vi "Filter by Favorites.vi"(8 "error in (no error)":errorcluster, 10 "Favorites? (T)":bool=TRUE, 11 "Contacts":T1[](array[typedef])) -> (0 "error out":errorcluster, 3 "Filtered Contacts":T1[](array[typedef]))   [LabVIEW 2014, in "Contact Data.lvlib"]
doc: "Filters an array of contacts to only include favorites or to not include favorites."
uses:
  Contact Data.lvlib
  Control Sort Mode.ctl
  Position.ctl
  Contact.ctl
  Controls.ctl
  DesinationControls.ctl
  DestinationCluster.ctl
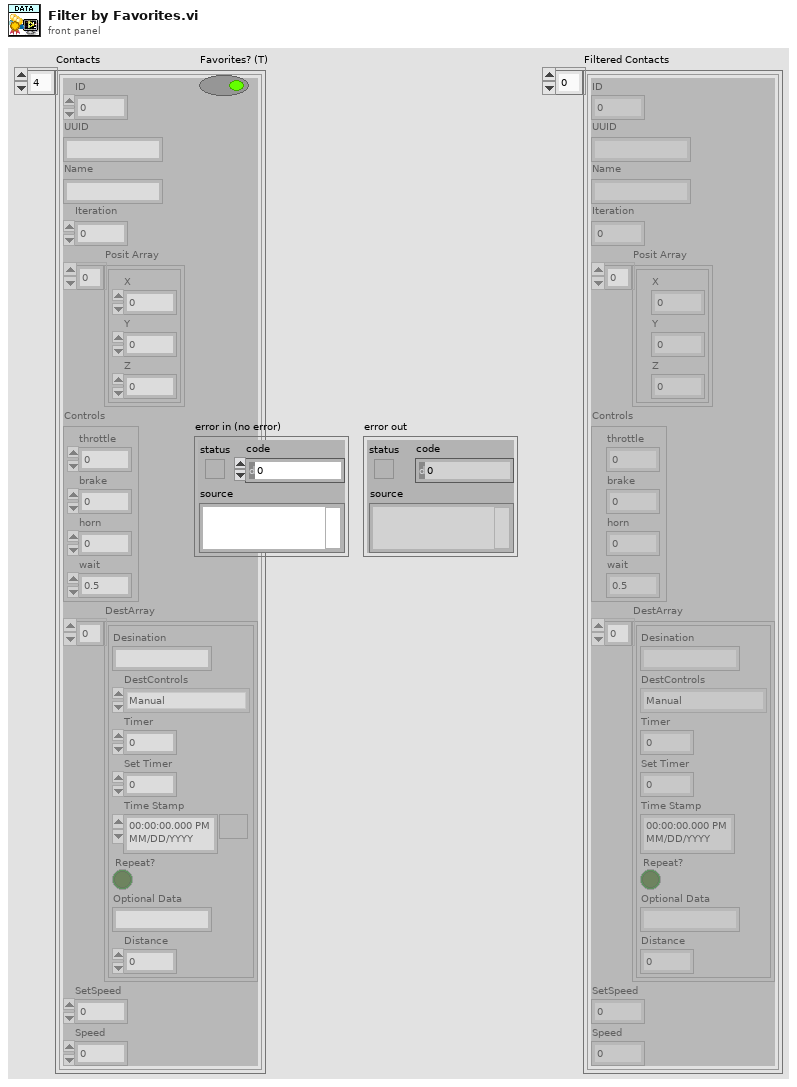
[diagram p1: front panel]
types:
  T1 = typedef "Contact Data.lvlib/Contact.ctl" = cluster{"ID":u32, "UUID":string, "Name":string, "Iteration":i32, "Posit Array":T2[], "Controls":T3, "DestArray":T4[], "SetSpeed":dbl, "Speed":dbl}
  T2 = typedef "Contact Data.lvlib/Position.ctl" = cluster{"X":dbl, "Y":dbl, "Z":dbl}
  T3 = typedef "Contact Data.lvlib/Controls.ctl" = cluster{"throttle":dbl, "brake":dbl, "horn":dbl, "wait":dbl}
  T4 = typedef "Contact Data.lvlib/DestinationCluster.ctl" = cluster{"Desination":string, "DestControls":T5, "Timer":u32, "Set Timer":u32, "Time Stamp":timestamp, "Repeat?":bool, "Optional Data":string, "Distance":dbl}
  T5 = typedef "Contact Data.lvlib/DesinationControls.ctl" = enum16{"Tracker", "Manual", "Stop", "Station DateTime", "Station Timer", "Maintain"}
  T6 = typedef "Contact Data.lvlib/Control Sort Mode.ctl" = u16
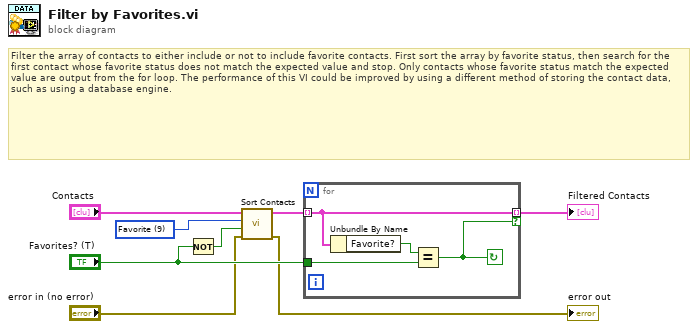
[diagram p0: block diagram]
diagram:
  w7 = T6 9 items=["Default", "Last Name", "First Name", "Middle Name", "Phone", "Street", "City", "State", "Postal Code", "Favorite"] ("Sort Mode (Default)")
  # "Filter the array of contacts to either include or not to include favorite contacts. First sort the array by favorite status, then search for the first contact whose favorite status does not match the expected value and stop. Only contacts whose favorite status match the expected value are output from the for loop. The performance of this VI could be improved by using a different method of storing the contact data, such as using a database engine."
  n1 = Not(x="Favorites? (T)") -> (.not. x?=w1:bool)
  n2 = call "Sort Contacts.vi"("error in (no error)"="error in (no error)", "Ascending? (T)"=w1, "Sort Mode (Default)"=w7, "Contacts"="Contacts") -> ("error out"=→"error out":errorcluster, "Sorted Contacts"=w4:T1[])  [unwired: 6 in]
  n3 = for {
    tunnel: w4 -> [w10] mode=indexing
    tunnel: "Favorites? (T)" -> [w11]
    tunnel: [w10] -> w2 mode=indexing if=w9
    stop <- w9 continue-if-true
    n4 = Unbundle By Name(w10) -> ("Favorite?"=w12:bool)
    n5 = Equal?(x=w12, y=w11) -> (x = y?=w9:bool)
  }
  "Filtered Contacts" <- w2
